vi "Faster Detector.vi"() -> ()   [LabVIEW 2018]
panel:
  out "XY Graph":cluster{dbl[], dbl[]}(graph)
  in  "velocity":dbl
  in  "bField":dbl
  in  "height":dbl
  in  "eField":dbl
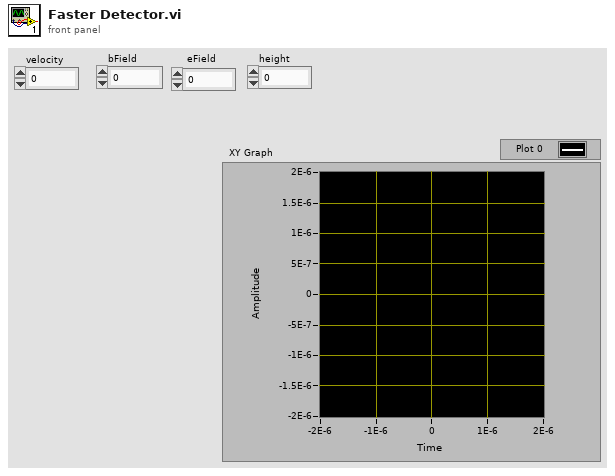
[diagram p1: front panel]
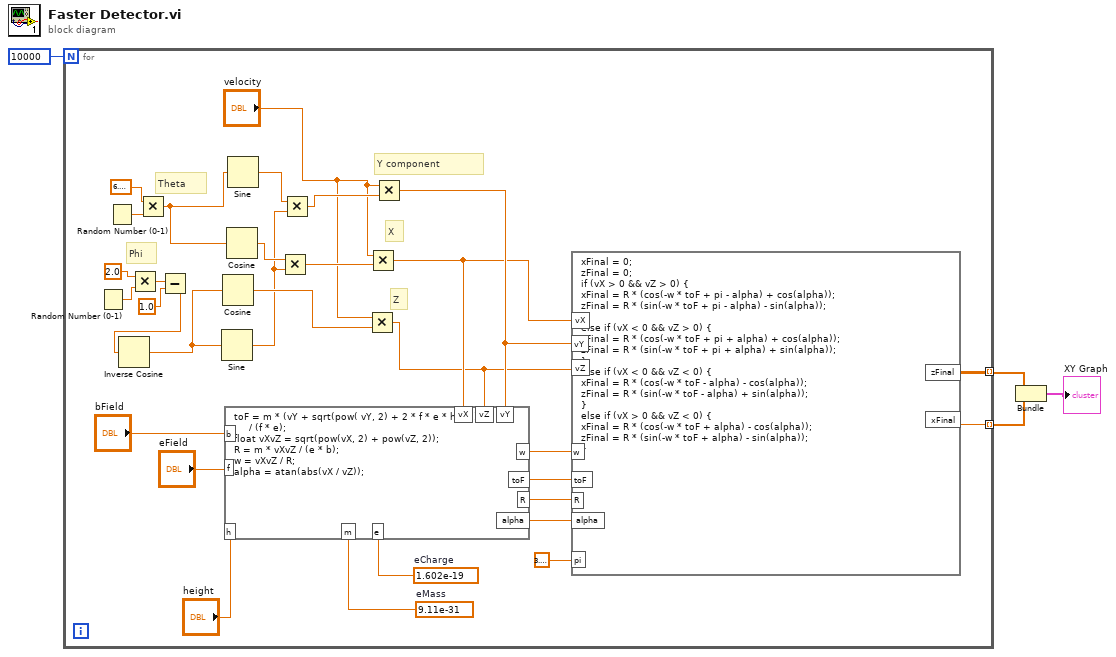
[diagram p0: block diagram]
diagram:
  n1 = for {
    N: 10000 -> [_]
    tunnel: [w7] -> w3 mode=indexing
    tunnel: [w6] -> w2 mode=indexing
    w33 = 1.602e-19  # eCharge
    w32 = 9.11e-31  # eMass
    # "Phi"
    # "Theta"
    # "Z"
    # "X"
    # "Y component"
    n2 = Random Number (0-1)() -> (number: 0 to 1=w27:dbl)
    n3 = Random Number (0-1)() -> (number: 0 to 1=w30:dbl)
    n4 = Multiply(x=2.0, y=w27) -> (x*y=w26:dbl)
    n5 = Multiply(x=6.283185307179586, y=w30) -> (x*y=w24:dbl)
    n6 = Subtract(x=w26, y=1.0) -> (x-y=w23:dbl)
    n7 = Inverse Cosine(1:w23) -> (0:w22:dbl)
    n8 = Sine(x=w22) -> (sin(x)=w17:dbl)
    n9 = Cosine(x=w22) -> (cos(x)=w21:dbl)
    n10 = Cosine(x=w24) -> (cos(x)=w18:dbl)
    n11 = Sine(x=w24) -> (sin(x)=w20:dbl)
    n12 = Multiply(x=w18, y=w17) -> (x*y=w16:dbl)
    n13 = Multiply(x=w20, y=w17) -> (x*y=w19:dbl)
    n14 = Multiply(x="velocity", y=w21) -> (x*y=w12:dbl)
    n15 = Multiply(x="velocity", y=w16) -> (x*y=w13:dbl)
    n16 = Multiply(x="velocity", y=w19) -> (x*y=w15:dbl)
    n17 = formula code="toF = m * (vY + sqrt(pow( vY, 2) + 2 * f * e * h / m))\n     / (f * e);\nfloat vXvZ = sqrt(pow(vX, 2) + pow(vZ, 2));\nR = m * vXvZ / (e * b);\nw = vXvZ / R;\nalpha = atan(abs(vX / vZ));"("f"="eField", "h"="height", "vY"=w15, "m"=w32, "e"=w33, "vX"=w13, "vZ"=w12, "b"="bField") -> ("toF"=w31:dbl, "w"=w11:dbl, "R"=w9:dbl, "alpha"=w8:dbl)
    n18 = formula code="xFinal = 0;\nzFinal = 0;\nif (vX > 0 && vZ > 0) {\nxFinal = R * (cos(-w * toF + pi - alpha) + cos(alpha));\nzFinal = R * (sin(-w * toF + pi - alpha) - sin(alpha));\n}\nelse if (vX < 0 && vZ > 0) {\nxFinal = R * (cos(-w * toF + pi + alpha) + cos(alpha));\nzFinal = R * (sin(-w * toF + pi + alpha) + sin(alpha));\n}\nelse if (vX < 0 && vZ < 0) {\nxFinal = R * (cos(-w * toF - alpha) - cos(alpha));\nzFinal = R * (sin(-w * toF - alpha) + sin(alpha));\n}\nelse if (vX > 0 && vZ < 0) {\nxFinal = R * (cos(-w * toF + alpha) - cos(alpha));\nzFinal = R * (sin(-w * toF + alpha) - sin(alpha));\n}"("vY"=w15, "toF"=w31, "vX"=w13, "vZ"=w12, "w"=w11, "R"=w9, "alpha"=w8, "pi"=3.141592653589793) -> ("zFinal"=w7:dbl, "xFinal"=w6:dbl)
  }
  n19 = Bundle(w3, w2) -> (→"XY Graph":cluster{dbl[], dbl[]})  [unwired: 1 in]
